vi "0-1 To OK-NG.vi"(11 "Result IN":string) -> (3 "Result Out":string)   [LabVIEW 2021]
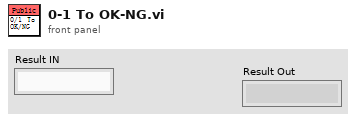
[diagram p1: front panel]
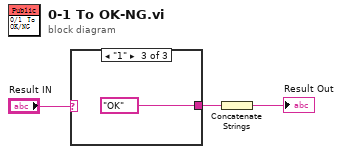
[diagram p0: block diagram]
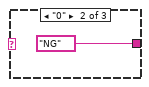
[diagram p3: hidden frame]
diagram:
  n1 = case shown="\"1\"" "Result IN" {
    selector: "Result IN" -> [w4 _ _]
    tunnel: [w4 "NG" ("Result") "OK" ("Result")] -> w2
    frame Default {
    }
    frame "0" {
    }
    frame "1" {
    }
  }
  n2 = Concatenate Strings(w2) -> (→"Result Out":string)
